vi "B_times_u.vi"(5 "Memory":refnum<k21>="Bz", 7 "NS":i16=5, 11 "u":sgl) -> (2 "product(vector)":sgl[](array[numeric]))   [LabVIEW 2017]
uses:
  <vilib>/Platform/TimedLoop/XDataNode/timing_clust.ctl
  <vilib>/Platform/TimedLoop/XDataNode/nitl_modes.ctl
  <vilib>/Platform/TimedLoop/XDataNode/wakeup.ctl
  <vilib>/rvi/Emulation/niFpgaSctlEmulationGetInTimedLoop.vi
  <vilib>/rvi/Emulation/niFpgaEmulationReportErrorSimple.vi
  <vilib>/rvi/Emulation/niFpgaGetClockAttributes.vi
  <vilib>/rvi/Emulation/niFpgaCriticalErrorInLSC.vi
  <vilib>/rvi/DataTransferAndStorage/Container/Common/niFpgaContainerExecOnDevCompGetState.vi
  <vilib>/rvi/Emulation/niFpgaEmulationIsFPGAContextNoSignature.vi
  <vilib>/rvi/DataTransferAndStorage/Container/Common/niFpgaContainerGetUniqueNameForEmu.vi
  <vilib>/rvi/Emulation/niFpgaProcessEmulError.vi
  <vilib>/rvi/errors/nirviReportUnexpectedCaseInternalError (U32).vi
  <vilib>/rvi/Memory/Memory_Emulation/niFpgaMemoryEmulationCacheClearOnFirstRun.vi
  <vilib>/rvi/Memory/Memory_Emulation/nirvimemoryEmulationManagerCache_MakeExclusive.vi
  <vilib>/rvi/Memory/Memory_Emulation/niFpgaMemoryEmulationValidateCache.vi
  <vilib>/rvi/Memory/Memory_Emulation/nirvimemoryEmulationManagerCache_InsertValue.vi
  <vilib>/Utility/error.llb/Clear Errors.vi
  <vilib>/rvi/Memory/Memory_Emulation/nirvimemoryEmulationManagerCache_ReleaseExclusive.vi
  <vilib>/rvi/Memory/Memory_Emulation/nirvimemoryEmulationManagerCache_GetValue.vi
  <vilib>/rvi/Memory/Memory_Emulation/nirvimemoryEmulationManagerCache_SetValue.vi
  <vilib>/rvi/Emulation/niFpgaSctlEmulationResourceMgr.vi
  <vilib>/Platform/TimedLoop/XDataNode/XDataNode.xnode
  <vilib>/rvi/DataTransferAndStorage/Container/XNode/niFpgaContainer.xnode
  <vilib>/rvi/Memory/Memory_Emulation/niFpgaMemoryEmulationRefIn.vi
  <vilib>/Platform/TimedLoop/XDataNode/XDNodeRunTimeDep.lvlib
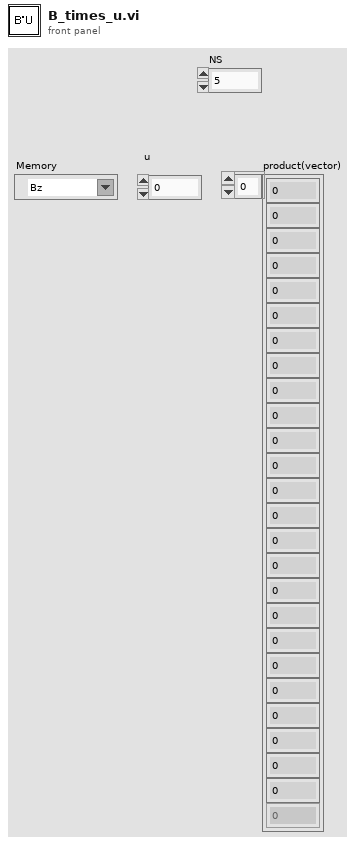
[diagram p1: front panel]
types:
  T1 = typedef "XDNodeRunTimeDep.lvlib/timing_clust.ctl" = cluster{"Expected End [f-1]":u64, "Actual End [f-1]":u64, "Finished Late? [f-1]":bool, "Expected End [i-1]":u64, "Actual End [i-1]":u64, "Finished Late? [i-1]":bool, "Expected Start [i]":u64, "Actual Start [i]":u64, "Expected Start [f]":u64, "Actual Start [f]":u64, "Source Name":string, "Structure Name":string, "Period":i64, "Deadline":i64, "Offset":i64, "Start":i64, "Priority":i32, "Timeout":i32, "Mode":T2, "Wakeup Reason":T3, "Error":errorcluster, "Source Type":string, "Secondary Source Type":string, "Global End Time":u64, "Global Start Time":u64, "Frame Duration":u64, "Iteration Duration":u64, "Assigned CPU":i32, "I/O Scan Engine Mode":u32}
  T2 = typedef "XDNodeRunTimeDep.lvlib/nitl_modes.ctl" = enum32{"No Change", "Process missed periods, maintain original phase", "Discard missed periods, maintain original phase", "Process missed periods, ignore original phase", "Discard missed periods, ignore original phase"}
  T3 = typedef "XDNodeRunTimeDep.lvlib/wakeup.ctl" = enum32{"Normal", "Aborted", "Asynchronous wakeup", "Timing source error", "Timed loop error", "Timeout"}
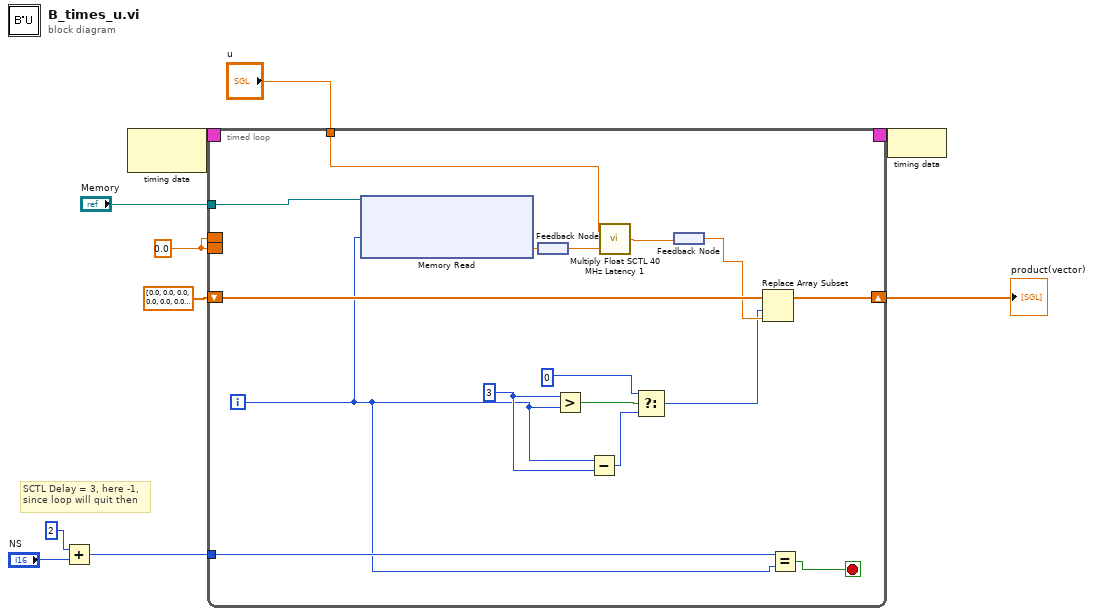
[diagram p0: block diagram]
diagram:
  w2 = sgl 0.0
  # "SCTL Delay = 3, here -1,\nsince loop will quit then"
  n1 = Add(x=i16 2, y="NS") -> (x+y=w5:i16)
  n2 = node-c288() -> (w10:T1)  [unwired: 1 in]
  n3 = timed-loop {
    timing: w10 -> [_]
    timing-out: [_] -> w9
    tunnel: "u" -> [w25]
    tunnel: w5 -> [w24]
    shift-right: [w22] -> w4
    shift-left: sgl[] [0.0, 0.0, 0.0, 0.0, 0.0, 0.0, 0.0, 0.0, 0.0, 0.0, 0.0, 0.0, 0.0, 0.0, 0.0, 0.0, 0.0, 0.0, 0.0, 0.0, 0.0, 0.0, 0.0, 0.0, 0.0] -> [w23]
    border: w2 -> [_]
    border: w2 -> [_]
    tunnel: "Memory" -> [w13]
    i -> [w11]
    stop <- w26 stop-if-true
    w14 = i16 3
    n4 = xnode ("Memory Read")("Address"=w11, "Memory In"=w13) -> ("Data"=w12:sgl)  [unwired: 1 out]
    n5 = feedback #1() -> (w15:sgl)
    n6 = feedback-in #1(w12) -> ()
    n7 = Greater?(x=w14, y=w11) -> (0:w16:bool)
    n8 = Subtract(x=w11, y=w14) -> (x-y=w18:i32)
    n9 = call "Multiply Float SCTL 40 MHz Latency 1.vi"("y"=w15, "x"=w25) -> ("x[k-1]*y[k-1]"=w21:sgl)
    n10 = Select(t=i16 0, s=w16, f=w18) -> (s? t:f=w17:i32)
    n11 = feedback-in #2(w21) -> ()
    n12 = feedback #2() -> (w20:sgl)
    n13 = Replace Array Subset(array=w23, new element=w20, index=w17) -> (w22:sgl[])
    n14 = Equal?(x=w24, y=w11) -> (x = y?=w26:bool)
  }
  "product(vector)" <- w4
  n15 = node-c288(w9) -> ()
